vi "Read_All_Reg.vi"(0 "Register":u16[](array[numeric]) format="%x", 1 "Slide Refnum":refnum<vi>, 2 "USB DAQ Address":i32 format="%x", 3 "Read I2C Address":u8 format="%x", 4 "Index to Reg No":u8[](array[numeric]) format="%x") -> (5 "Output Register":u16[](array[numeric]) format="%x", 6 "Status":string="ERROR COMMUNICATING WITH DEVICE")   [LabVIEW 2011]
doc: "This VI is used to read all registers of a device, using the TMP101 as a template. The existing register array, the device address, and I2C device address are sent to the \"Read Single Reg\" VI which converts and concatenates the inputs into a mnemonic command which is then sent to the \"RunMnemCmd\" VI. The VI outputs the results of the reads and also performs error-checks on the ACKS arrays. If an error is found, the VI reports to Main and displays an error message."
panel:
  out "Comm Error Flags":bool[](array[boolean])
  out "Status String Array":string[](array[string])
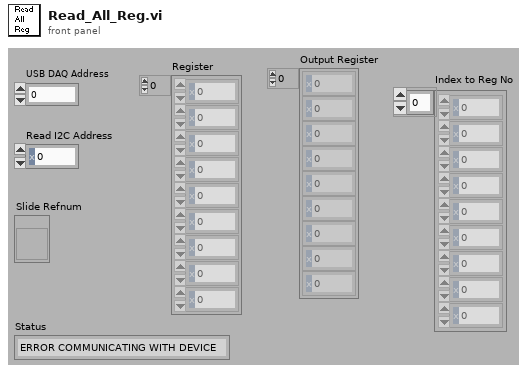
[diagram p1: front panel]
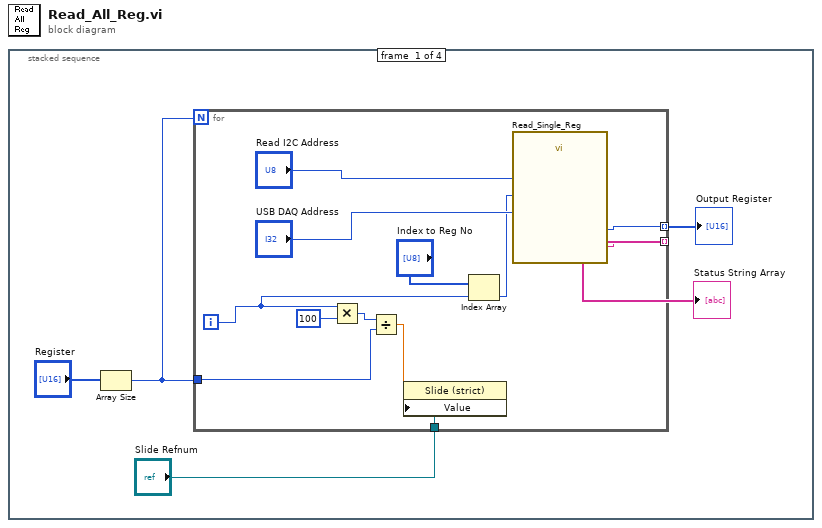
[diagram p0: block diagram]
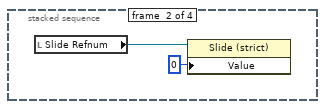
[diagram p2: hidden frame]
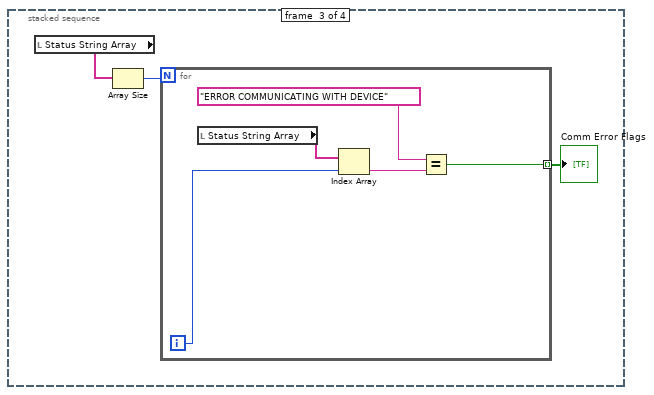
[diagram p3: hidden frame]
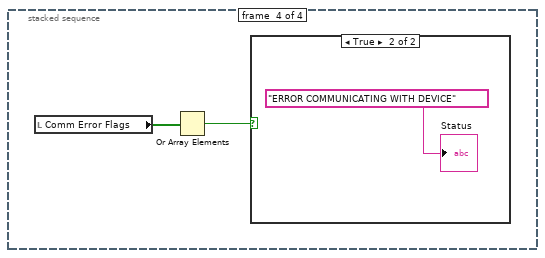
[diagram p4: hidden frame]
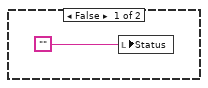
[diagram p5: hidden frame]
diagram:
  n1 = stacked-sequence {
    frame #0 {
      n2 = Array Size(array="Register") -> (size(s)=w2:i32)
      n3 = for {
        N: w2 -> [_]
        tunnel: [w17] -> w5 mode=indexing
        tunnel: "Slide Refnum" -> [w11]
        tunnel: w2 -> [w10]
        tunnel: [w9] -> w1 mode=indexing
        i -> [w6]
        n4 = Multiply(x=w6, y=100) -> (x*y=w14:i32)
        n5 = Divide(x=w14, y=w10) -> (x/y=w13:dbl)
        n6 = property class="Slide (strict)"(reference=w11, "Value"=w13) -> ()  [unwired: 1 in, 2 out]
        n7 = Index Array(array="Index to Reg No", index=w6) -> (element=w8:u8)
        n8 = call "Read_Single_Reg.vi"("Read I2C Address"="Read I2C Address", "USB DAQ Address"="USB DAQ Address", "Reg No"=w8) -> ("Status String"=w9:string, "Read Result"=w17:u16)
      }
      "Output Register" <- w5
      "Status String Array" <- w1
    }
    frame #1 {
      n9 = local read "Slide Refnum"() -> (w18:refnum<vi>)
      n10 = property class="Slide (strict)"(reference=w18, "Value"=u8 0) -> ()  [unwired: 1 in, 2 out]
    }
    frame #2 {
      n11 = local read "Status String Array"() -> (w20:string[])
      n12 = Array Size(array=w20) -> (size(s)=w21:i32)
      n13 = for {
        N: w21 -> [_]
        tunnel: [w24] -> w22 mode=indexing
        i -> [w27]
        n14 = local read "Status String Array"() -> (w23:string[])
        n15 = Index Array(array=w23, index=w27) -> (element=w26:string)
        n16 = Equal?(x="ERROR COMMUNICATING WITH DEVICE", y=w26) -> (x = y?=w24:bool)
      }
      "Comm Error Flags" <- w22
    }
    frame #3 {
      n17 = local read "Comm Error Flags"() -> (w29:bool[])
      n18 = Or Array Elements(Boolean array=w29) -> (logical OR=w28:bool)
      n19 = case shown="True" w28 {
        frame False {
          n20 = local write "Status"("") -> ()
        }
        frame True {
          "Status" <- "ERROR COMMUNICATING WITH DEVICE"
        }
      }
    }
  }
